vi "Read Behavior.vi"(11 "Flex Dialog in":refnum<class "Flex UI Dialog.lvclass">) -> (2 "Behavior":T1(ring)=enum."Default", 3 "Flex Dialog out":refnum<class "Flex UI Dialog.lvclass">)   [LabVIEW 2016, in "Flex UI Dialog.lvclass"]
uses:
  Flex UI Dialog.lvclass
  Flex UI Dialog.lvclass/Flex UI Dialog.ctl
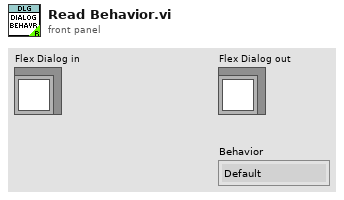
[diagram p1: front panel]
types:
  T1 = enum32{"Invalid", "Default", "Floating", "Floating/Auto-Hide", "Modal"}
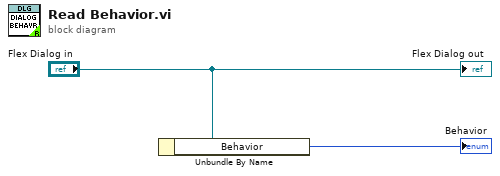
[diagram p0: block diagram]
diagram:
  n1 = Unbundle By Name("Flex Dialog in") -> ("Behavior"=→"Behavior":T1)
  "Flex Dialog out" <- "Flex Dialog in"
